vi "Clear Setup Display.vi"(8 "error in (no error)":errorcluster, 11 "UI in":refnum<class "UI.lvclass">) -> (0 "error out":errorcluster)   [LabVIEW 2020, in "AR Example.lvlib" / "UI.lvclass"]
uses:
  UI.lvclass
  UI.lvclass/UI.ctl
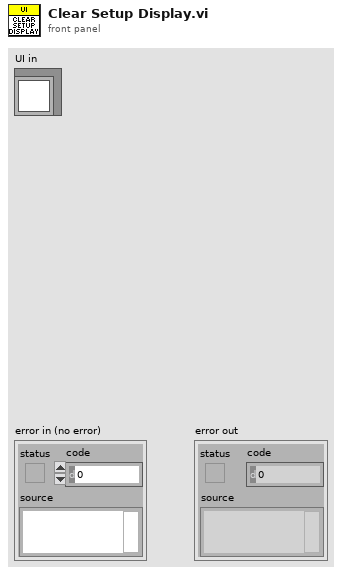
[diagram p1: front panel]
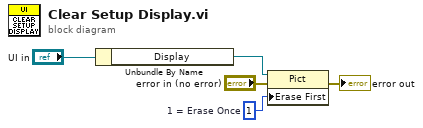
[diagram p0: block diagram]
diagram:
  w3 = u8 1  # 1 = Erase Once
  n1 = Unbundle By Name("UI in") -> ("Display"=w4:refnum<vi>)
  n2 = property class="Pict"(reference=w4, error in="error in (no error)", "Erase First"=w3) -> (error out=→"error out":errorcluster)  [unwired: 1 out]
